vi "GEOM_Size2Coords.vi"(10 "Size":T1) -> (2 "Coords":T2)   [LabVIEW 2016]
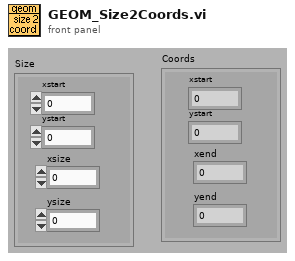
[diagram p1: front panel]
types:
  T1 = cluster{"xstart":i32, "ystart":i32, "xsize":i32, "ysize":i32}
  T2 = cluster{"xstart":i32, "ystart":i32, "xend":i32, "yend":i32}
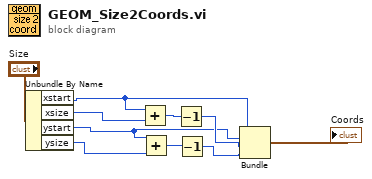
[diagram p0: block diagram]
diagram:
  n1 = Unbundle By Name("Size") -> ("xstart"=w5:i32, "xsize"=w4:i32, "ystart"=w3:i32, "ysize"=w2:i32)
  n2 = Add(x=w5, y=w4) -> (x+y=w10:i32)
  n3 = Add(x=w3, y=w2) -> (x+y=w9:i32)
  n4 = Decrement(x=w10) -> (x-1=w8:i32)
  n5 = Decrement(x=w9) -> (x-1=w7:i32)
  n6 = Bundle("xstart"=w5, "ystart"=w3, w8, w7) -> (→"Coords":cluster{"xstart":i32, "ystart":i32, i32, i32})  [unwired: 1 out]
